vi "GOLPI full test - part test vector complex.vi"(6 "column vector?":bool, 7 "set: use temporary file?":bool, 8 "error in (no error)":errorcluster, 9 "test value":cdb[](array[numeric])=[1.234+0.0i, 2.345+0.0i, 3.456+0.0i], 10 "variable name in":string, 11 "GOLPI ref. in":T1) -> (0 "error out":errorcluster, 2 "test result":bool, 3 "GOLPI ref. out":T1)   [LabVIEW 2013]
uses:
  Private/Type Definitions/GOLPI reference Type Def.ctl
  LV Process.lvlibp/Pipe Handle.ctl
  Private/Set Variable - polymorph parts/Set 1D Array Double Complex.vi
  Private/Get Variable - polymorph parts/Get 1D Array Double Complex.vi
  GOLPI library.lvlib
  LV Process.lvlibp
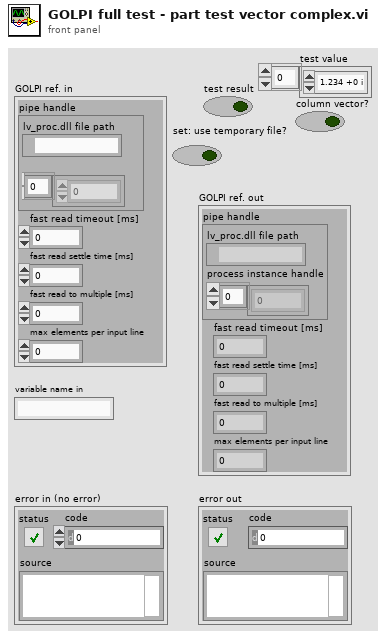
[diagram p1: front panel]
types:
  T1 = typedef "GOLPI library.lvlib/GOLPI reference Type Def.ctl" = cluster{"pipe handle":T2, "fast read timeout [ms]":u32, "fast read settle time [ms]":u32, "fast read to multiple [ms]":u32, "max elements per input line":u32}
  T2 = typedef "LV Process.lvlibp/Pipe Handle.ctl" = cluster{"lv_proc.dll file path":path, "process instance handle":u32[]}
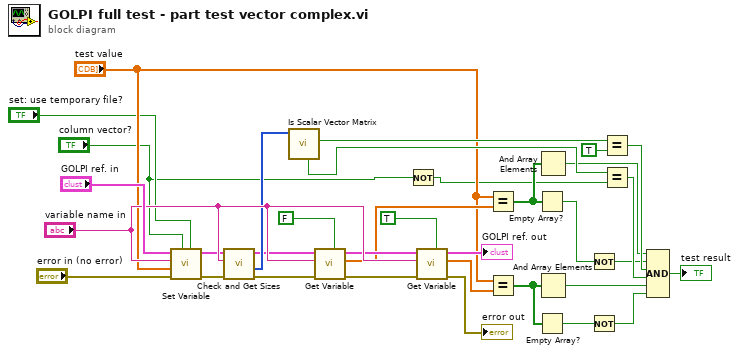
[diagram p0: block diagram]
diagram:
  n1 = call-poly "Set Variable.vi"("use temporary file?"="set: use temporary file?", "column vector?"="column vector?", "error in"="error in (no error)", "value"="test value", "variable name"="variable name in", "GOLPI ref. in"="GOLPI ref. in") -> ("error out"=w10:errorcluster, "GOLPI ref. out"=w11:T1)  [unwired: 4 in]
  n2 = call "Check and Get Sizes.vi"("error in (no error)"=w10, "variable name"="variable name in", "GOLPI ref. in"=w11) -> ("error out"=w13:errorcluster, "octave sizes"=w14:i32[], "GOLPI ref. out"=w12:T1)  [unwired: 5 in, 1 out]
  n3 = call "Is Scalar Vector Matrix.vi"("octave sizes"=w14) -> ("is vector?"=w18:bool, "row vector?"=w15:bool)  [unwired: 5 in, 4 out]
  n4 = call-poly "Get Variable.vi"("use temporary file?"=FALSE, "error in"=w13, "variable name"="variable name in", "GOLPI ref. in"=w12) -> ("error out"=w21:errorcluster, "value"=w9:cdb[], "GOLPI ref. out"=w20:T1)  [unwired: 5 in]
  n5 = Not(x="column vector?") -> (.not. x?=w1:bool)
  n6 = call-poly "Get Variable.vi"("use temporary file?"=TRUE, "error in"=w21, "variable name"="variable name in", "GOLPI ref. in"=w20) -> ("error out"=→"error out":errorcluster, "value"=w26:cdb[], "GOLPI ref. out"=→"GOLPI ref. out":T1)  [unwired: 5 in]
  n7 = Equal?(x="test value", y=w9) -> (x = y?=w8:bool[])
  n8 = Equal?(x="test value", y=w26) -> (x = y?=w24:bool[])
  n9 = Empty Array?(array=w8) -> (empty?=w7:bool)
  n10 = Empty Array?(array=w24) -> (empty?=w25:bool)
  n11 = And Array Elements(Boolean array=w8) -> (logical AND=w5:bool)
  n12 = And Array Elements(Boolean array=w24) -> (logical AND=w27:bool)
  n13 = Not(x=w7) -> (.not. x?=w6:bool)
  n14 = Not(x=w25) -> (.not. x?=w28:bool)
  n15 = Equal?(x=w18, y=TRUE) -> (x = y?=w19:bool)
  n16 = Equal?(x=w15, y=w1) -> (x = y?=w16:bool)
  n17 = Compound Arithmetic op=AND(w5, w6, w19, w16, w27, w28) -> (→"test result":bool)
